vi "runAbsorptionAnalysis.vi"(8 "error in (no error)":errorcluster, 11 "ImageStreamViewer in":refnum<class "ImageStreamViewer.lvclass">) -> (0 "error out":errorcluster, 3 "ImageStreamViewer out":refnum<class "ImageStreamViewer.lvclass">)   [LabVIEW 2011, in "Views.lvlib" / "Camera.lvlib" / "ImageStreamViewer.lvclass"]
uses:
  ImageStreamViewer.lvclass
  Tools/ImageProcessor/ImageAnalyser/AbsorptionAnalyser/AbsorptionAnalyser.lvclass
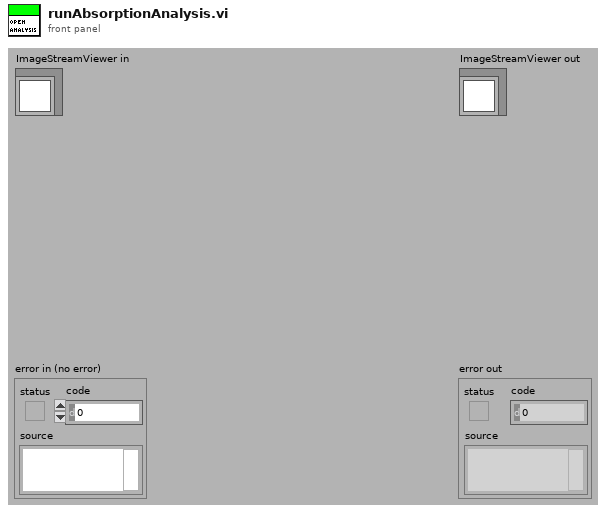
[diagram p1: front panel]
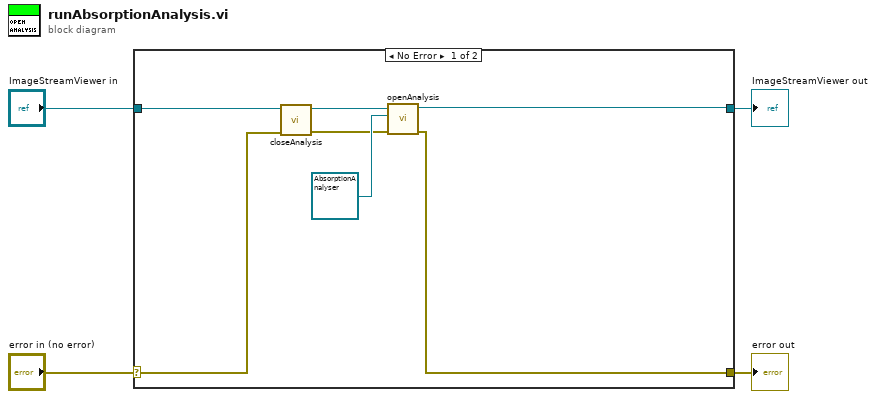
[diagram p0: block diagram]
diagram:
  n1 = case shown="No Error" "error in (no error)" {
    selector: "error in (no error)" -> [w5 w13]
    tunnel: [w10 w13] -> w3
    tunnel: [w11 w12] -> w1
    tunnel: "ImageStreamViewer in" -> [w8 w12]
    frame No Error {
      n2 = call "closeAnalysis.vi"("error in (no error)"=w5, "ImageStreamViewer in"=w8) -> ("error out"=w6:errorcluster, "ImageStreamViewer out"=w7:refnum<class "ImageStreamViewer.lvclass">)  [unwired: 8 in]
      n3 = call "openAnalysis.vi"("error in (no error)"=w6, "ImageAnalyser"=refnum<class "AbsorptionAnalyser.lvclass"> refnum ("Tools.lvlib:Imaging.lvlib:AbsorptionAnalyser.lvclass"), "ImageStreamViewer in"=w7) -> ("error out"=w10:errorcluster, "ImageStreamViewer out"=w11:refnum<class "ImageStreamViewer.lvclass">)  [unwired: 7 in]
    }
    frame Error {
    }
  }
  "error out" <- w3
  "ImageStreamViewer out" <- w1
